vi "TAT_Start.vi"(8 "error In":errorcluster) -> (0 "error out":errorcluster)   [LabVIEW 2017]
uses:
  <vilib>/Utility/error.llb/DialogType.ctl
  Controls/Ass. Loop Control.ctl
  <vilib>/addons/database/Connection.llb/Conn ObjectReference.ctl
  227c0874-5cf7-40bb-b9d2-311cfb67fe7f.vi
  Global/Global 1.vi
  <vilib>/Instr/_visa.llb/VISA Configure Serial Port (Instr).vi
  <vilib>/addons/database/NI_Database_API.lvlib
  <vilib>/Utility/config.llb/NI_LVConfig.lvlib
panel:
  out "12 4":bool
  out "EOL AUTO CYCLE STATUS:-":bool
  out "12 3":bool
  out "12 2":bool
  out "12":bool
  out "PLC STATUS:-":bool
  out "array":string[](array[string])
  out "LEAK UNIT RESULT 2":bool caption="LEAK RESULT:-"
  out "LEAK ACTUAL VALUE 2":string
  out "LEAK MAX 2":string
  out "LEAK MIN 2":string
  out "LEAK UNIT RESULT":bool caption="LEAK RESULT:-"
  out "LEAK ACTUAL VALUE":string
  out "LEAK MAX":string
  out "LEAK MIN":string
  out "PREVIOUS BARCODE":string[](array[string])
  out "scanned":string
  out "Scanned Qyt":string
  out "PROJECT :-":string
  out "PACKAGE Qty":string
  out "TORISHI CODE:-":string
  out "PART No.:-":string
  in  "Stop":bool
  out "BARCODE STATION 2":string caption="BARCODE:-"
  out "RESULT STATION 1":bool caption="FINAL RESULT:-"
  out "USER:-":string
  out "PART NAME :-":string
  in  "ASS-Alarms":bool
  out "CYCLE STATUS STATION 1":string caption="CYCLE STATUS:-"
  out "DATE/TIME":string
  # "KAPSE SONS ROBOTICS\n& AUTOMATION"
  # "Nm"
  # "POKA-YOKE STATUS"
  # "LEAK TESTING PARAMETER"
  # "MIN"
  # "MAX"
  # "ACTUAL VALUE"
  # "RESULT"
  # "LEAK UNIT"
  # "LEAK PRESSURE"
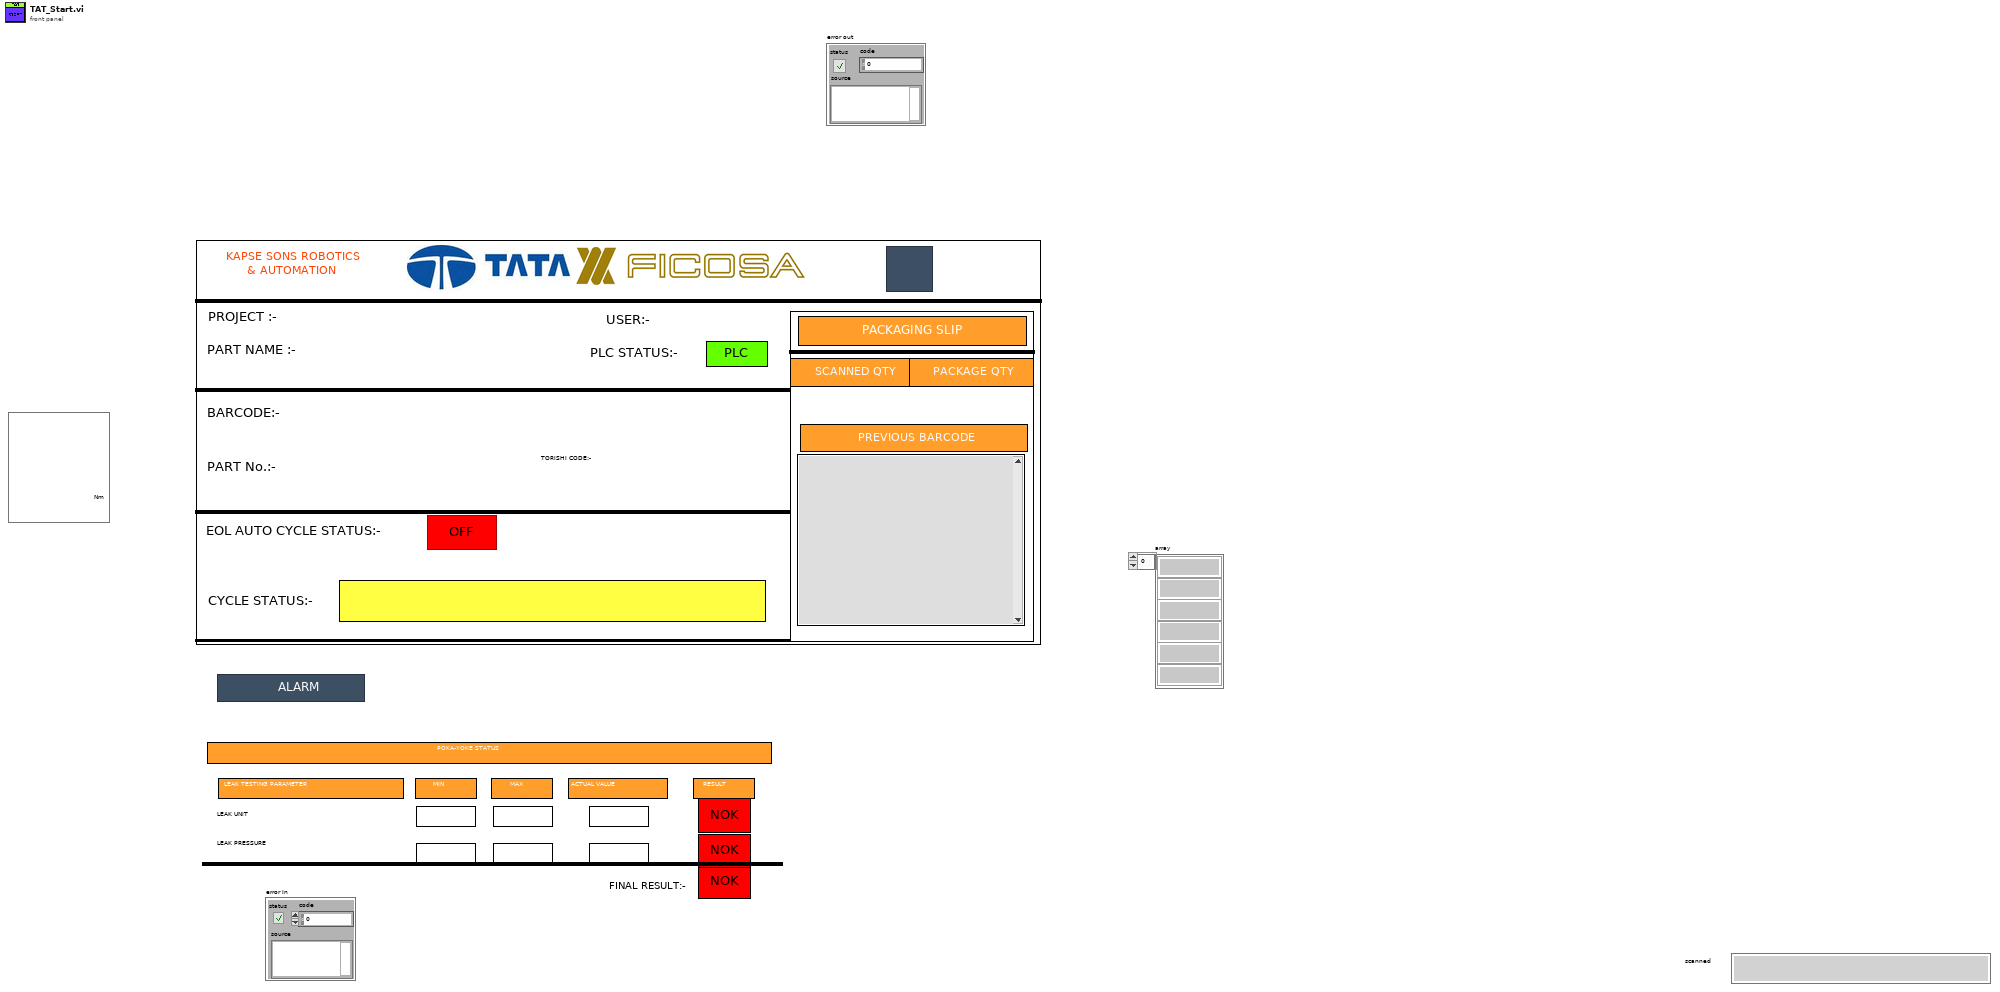
[diagram p1: front panel]
types:
  T1 = typedef "NI_Database_API.lvlib/Conn ObjectReference.ctl" = refnum<k1>
  T2 = cluster{"Varient number":u16, "Part name":string, "Barcode":string, "connection reference":T1, "Batch_Size":u16, "PART_NO":string, "TORISHI_CODE":string, "scanner com":refnum<visa-resource-name>, "Part Name List":string[], "Varient path":path, "Current Varient path":path, "Communication path":path, "PRN path":path, "printer":refnum<k5>, "Data_log_Path":path, "PREVIOUS Code":string[], "Printer IP add":string}
  T3 = typedef "Ass. Loop Control.ctl" = enum16{"Int2", "Package_Qty_Count", "GENERATE_QR_PRNT", "Cluster_update", "Waiting_for_scan", "barcode CHECK", "Int", "SaveReport ", "Barcode Print", "Start Cycle", "Wait", "Cycle End", "Stop"}
  T4 = typedef "DialogType.ctl" = u16
  T5 = enum32{"invalid app kind", "Development System", "Run Time System", "Student Edition", "Embedded LabVIEW", "Evaluation", "Custom"}
  T6 = typedef "NI_LVConfig.lvlib/Config Data RefNum.ctl" = refnum<k1>
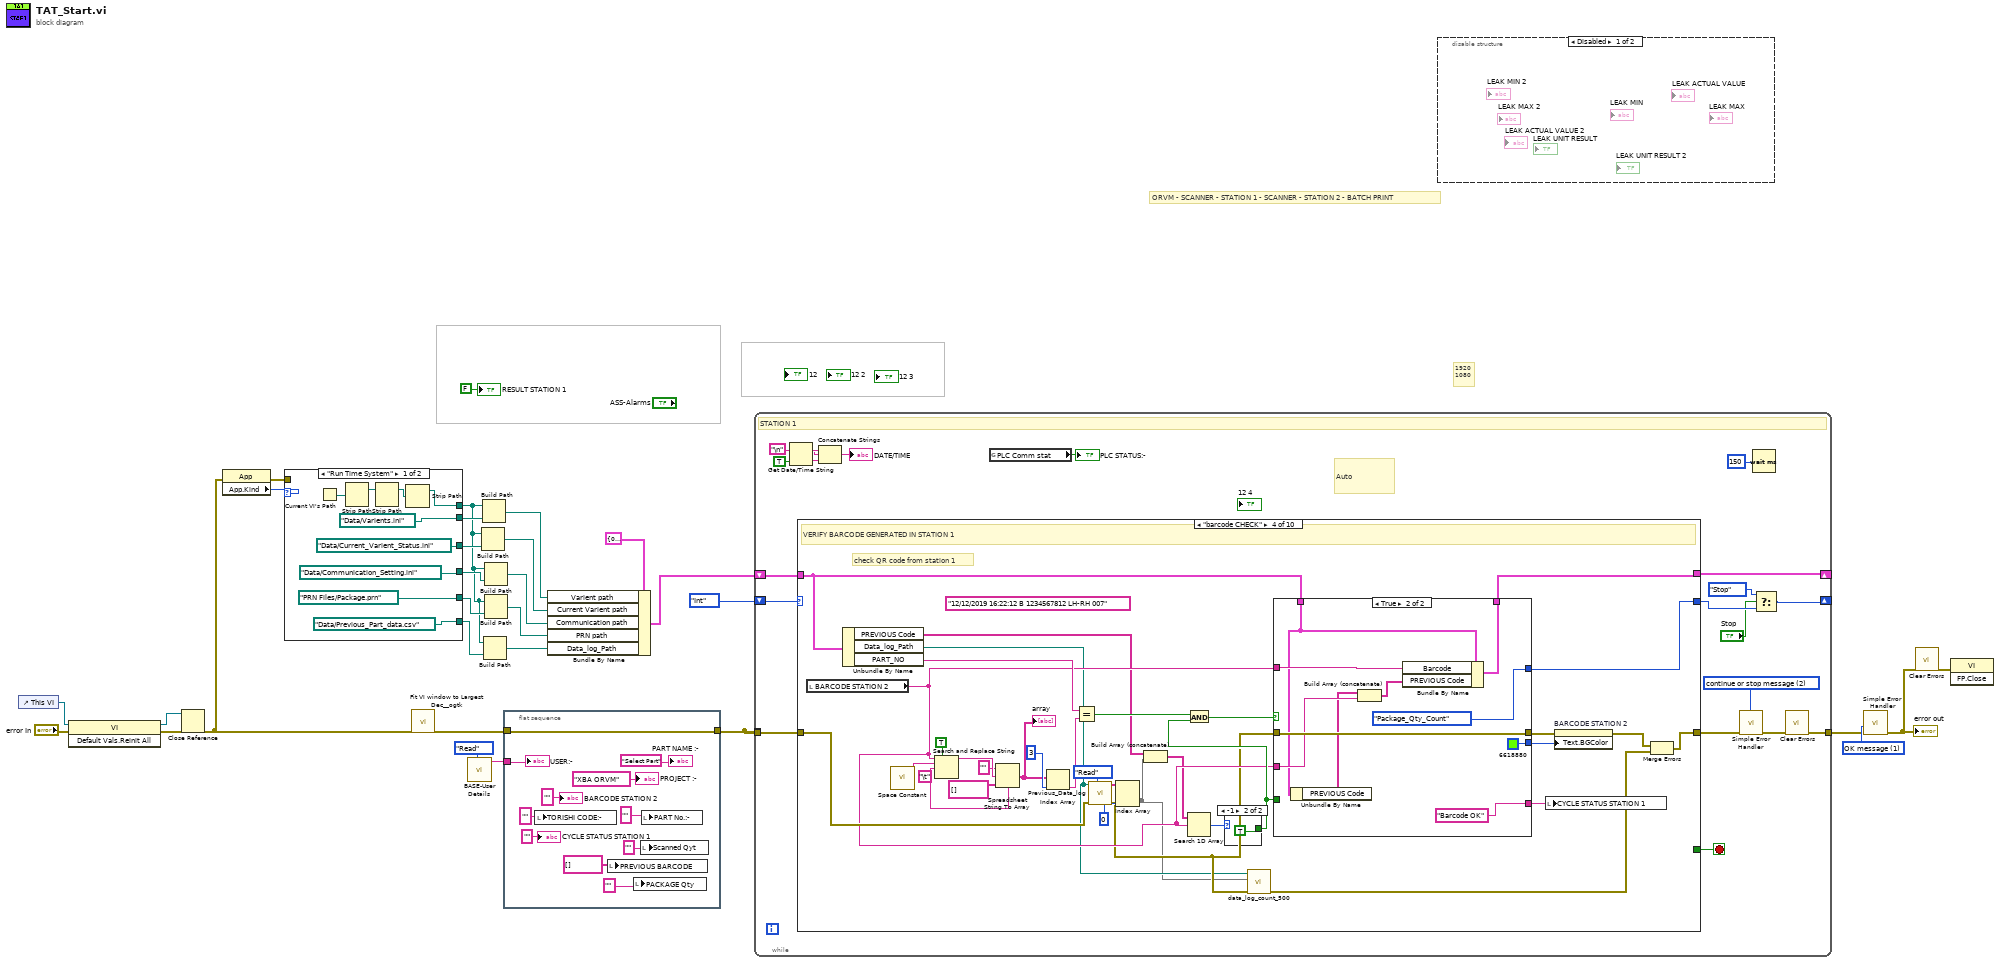
[diagram p0: block diagram]
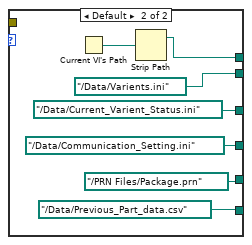
[diagram p2: hidden frame]
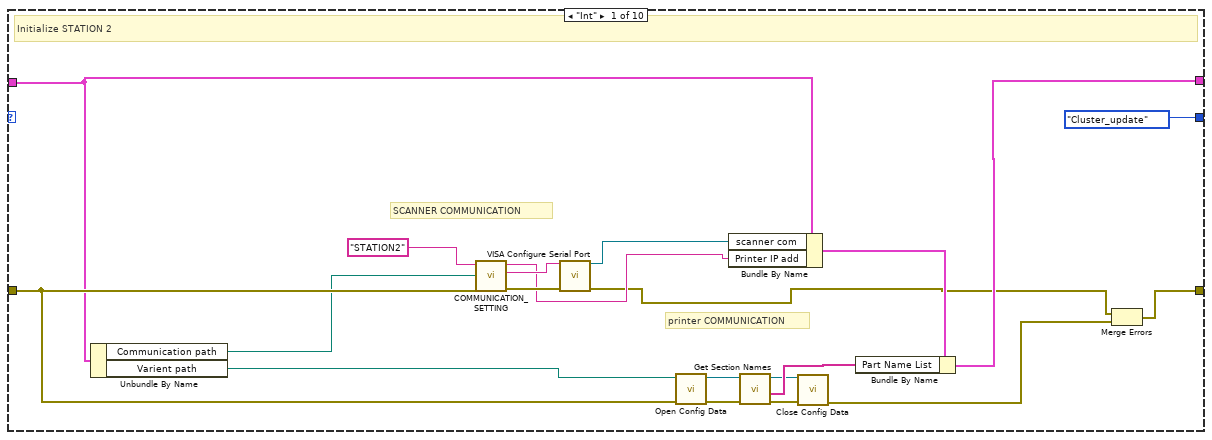
[diagram p4: hidden frame]
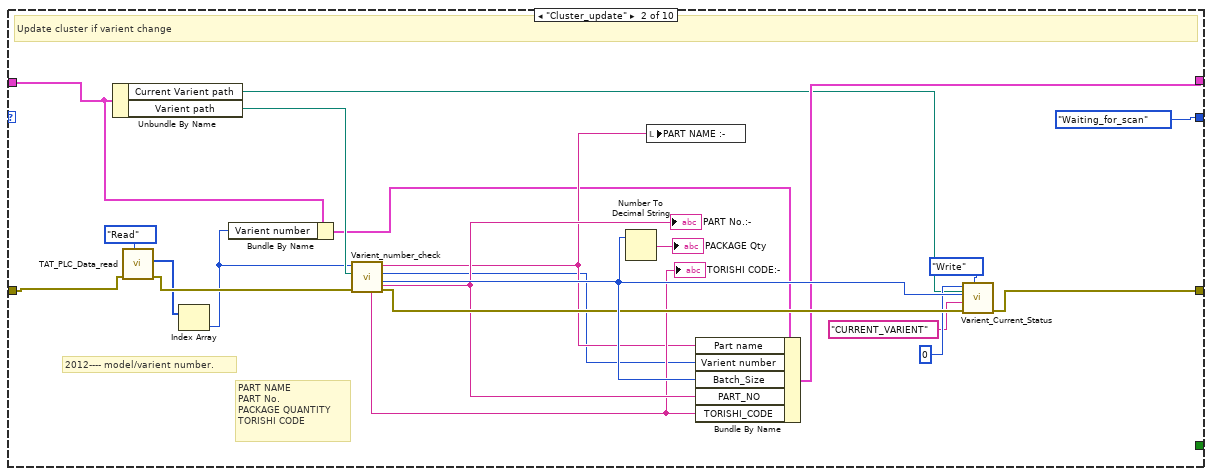
[diagram p5: hidden frame]
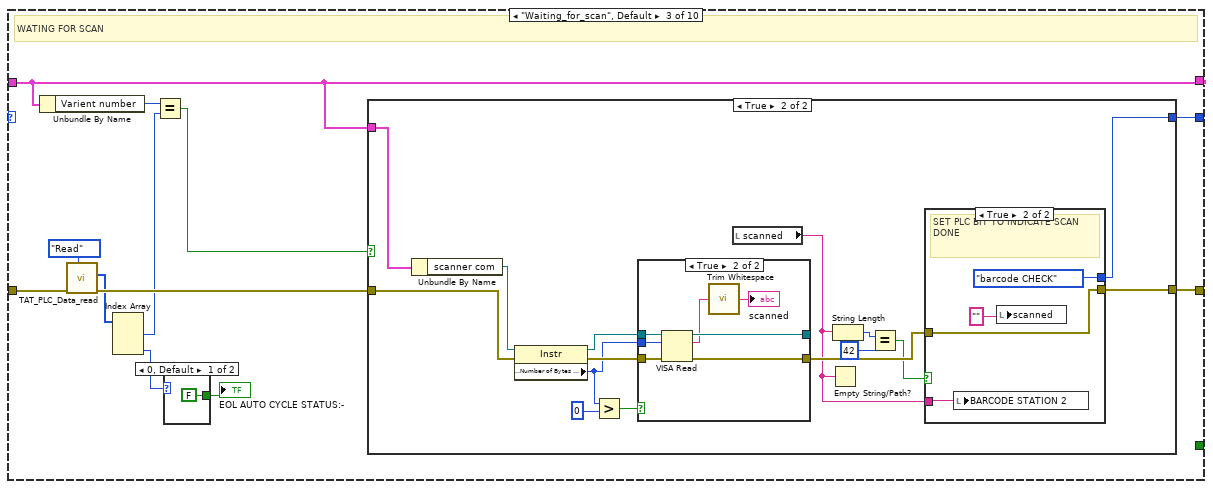
[diagram p6: hidden frame]
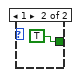
[diagram p7: hidden frame]
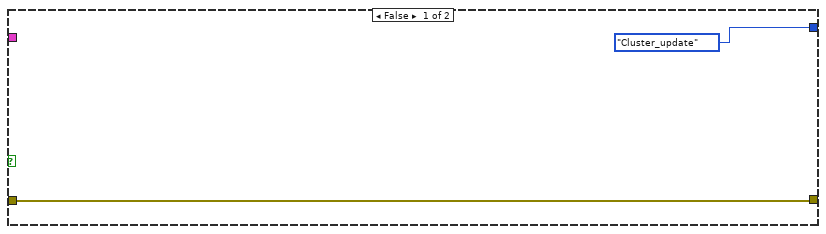
[diagram p8: hidden frame]
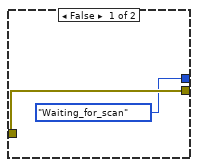
[diagram p10: hidden frame]
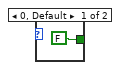
[diagram p11: hidden frame]
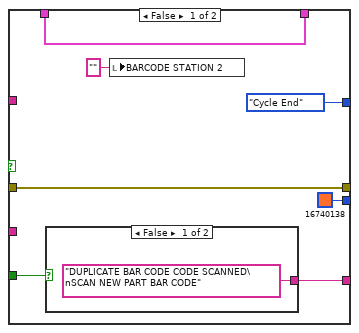
[diagram p12: hidden frame]
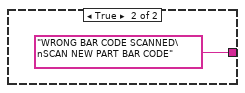
[diagram p13: hidden frame]
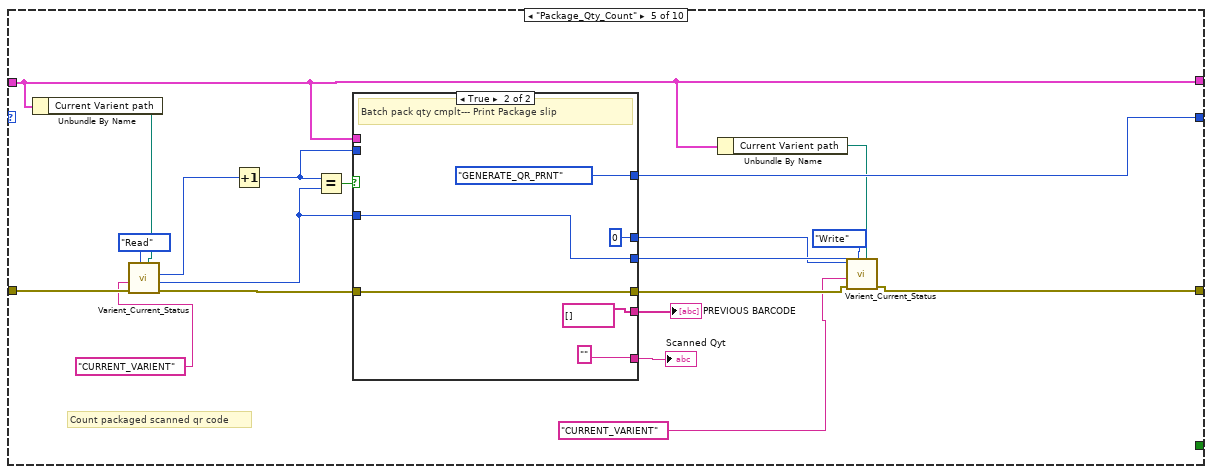
[diagram p14: hidden frame]
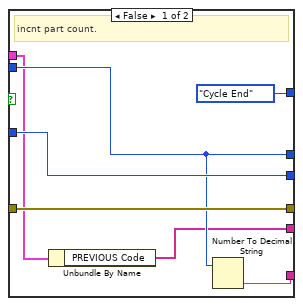
[diagram p15: hidden frame]
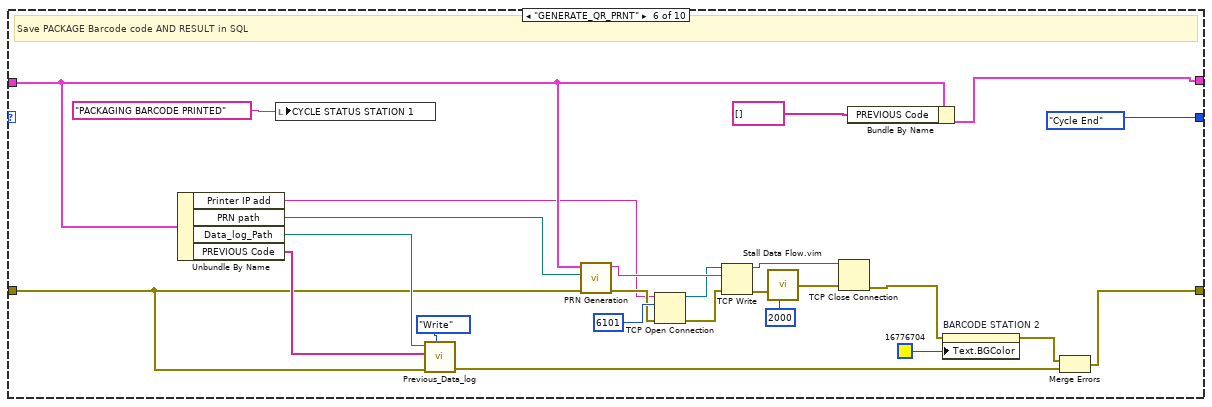
[diagram p16: hidden frame]
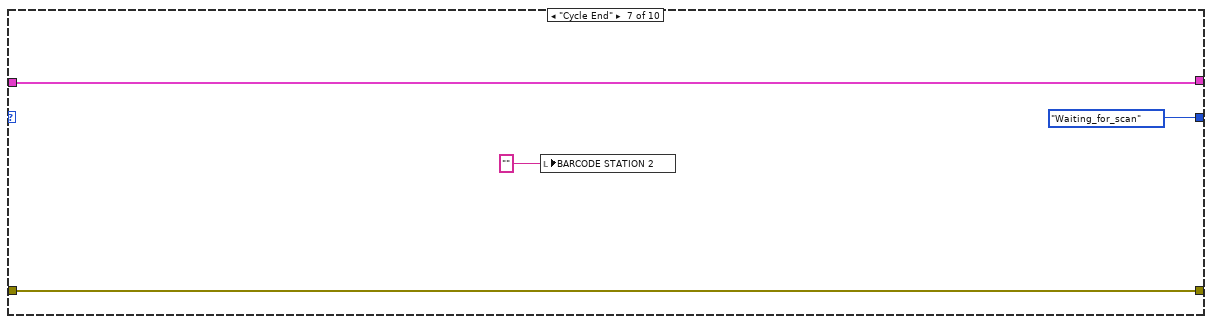
[diagram p17: hidden frame]
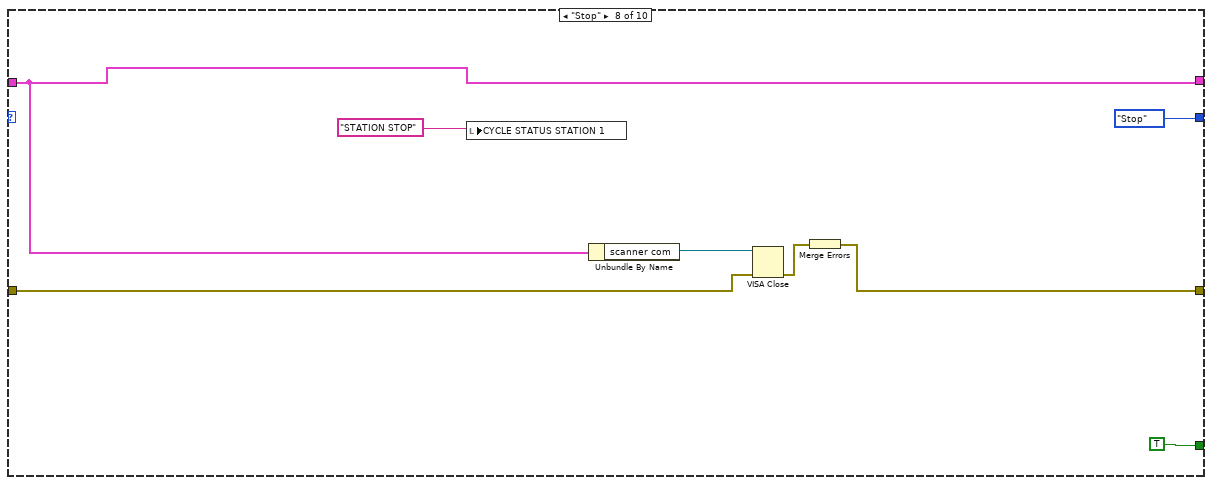
[diagram p18: hidden frame]
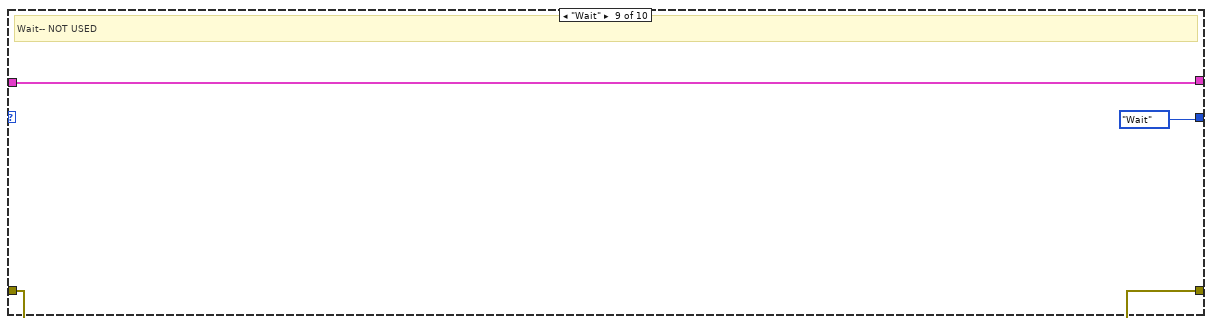
[diagram p19: hidden frame]
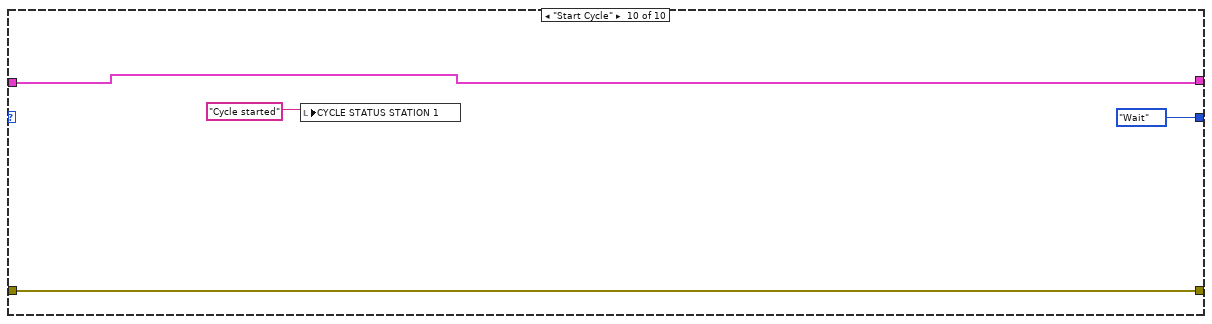
[diagram p20: hidden frame]
diagram:
  w20 = T4 1 items=["no dialog", "OK message", "continue or stop message", "OK message + warnings", "continue/stop + warnings"] ("type of dialog (OK msg:1)")
  # "1920\n1080"
  # "ORVM - SCANNER - STATION 1 - SCANNER - STATION 2 - BATCH PRINT"
  n1 = control-ref of="This VI"() -> (w30:refnum<vi>)
  n2 = invoke class="VI" method="Default Vals.Reinit All"(reference=w30, error in="error In") -> (reference out=w27:refnum<vi>, error out=w28:errorcluster)  [unwired: 1 in, 1 out]
  n3 = Close Reference(reference=w27, error in (no error)=w28) -> (error out=w4:errorcluster)
  n4 = property class="App"(error in=w4) -> (error out=w7:errorcluster, "App.Kind"=w16:T5)  [unwired: 1 in, 1 out]
  n5 = case shown="\"Run Time System\"" w16 {
    tunnel: [path "Data/Varients.ini" ("path") path "../Data/Varients.ini" ("path")] -> w15
    tunnel: [w35 w44] -> w5
    tunnel: [path "Data/Current_Varient_Status.ini" ("path") path "../Data/Current_Varient_Status.ini" ("path")] -> w12
    tunnel: [path "Data/Communication_Setting.ini" ("path") path "../Data/Communication_Setting.ini" ("path")] -> w11
    tunnel: [path "PRN Files/Package.prn" ("path") path "../PRN Files/Package.prn" ("path")] -> w9
    tunnel: w7 -> [_ _]
    tunnel: [path "Data/Previous_Part_data.csv" ("path") path "../Data/Previous_Part_data.csv" ("path")] -> w1
    frame "Run Time System" {
      n6 = Current VI's Path() -> (path=w38:path)
      n7 = Strip Path(path=w38) -> (stripped path=w37:path)  [unwired: 1 out]
      n8 = Strip Path(path=w37) -> (stripped path=w36:path)  [unwired: 1 out]
      n9 = Strip Path(path=w36) -> (stripped path=w35:path)  [unwired: 1 out]
    }
    frame Default {
      n10 = Current VI's Path() -> (path=w45:path)
      n11 = Strip Path(path=w45) -> (stripped path=w44:path)  [unwired: 1 out]
    }
  }
  n12 = call <userlib>:"Fit VI window to Largest Dec__ogtk.vi"("error in (no error)"=w4) -> ("error out"=w26:errorcluster)  [unwired: 5 in, 1 out]
  n13 = call "BASE-User Details.vi"("Enum"=enum16{"Read", "Write"}."Read") -> ("User Name Out"=w21:string)  [unwired: 9 in, 1 out]
  n14 = Build Path(base path=w5, name or relative path=w12) -> (appended path=w13:path)
  n15 = Build Path(base path=w5, name or relative path=w15) -> (appended path=w14:path)
  n16 = Build Path(base path=w5, name or relative path=w1) -> (appended path=w6:path)
  n17 = Build Path(base path=w5, name or relative path=w11) -> (appended path=w10:path)
  n18 = Build Path(base path=w5, name or relative path=w9) -> (appended path=w8:path)
  n19 = flat-sequence {
    tunnel: [w57] -> w18
    tunnel: w26 -> [w57]
    tunnel: w21 -> [w56]
    frame #0 {
      n20 = local write "TORISHI CODE:-"("") -> ()
      n21 = local write "PREVIOUS BARCODE"(string[] []) -> ()
      n22 = local write "PACKAGE Qty"("") -> ()
      n23 = local write "Scanned Qyt"("") -> ()
      n24 = local write "PART No.:-"("") -> ()
      "USER:-" <- w56
      "PART NAME :-" <- "Select Part"
      "PROJECT :-" <- "XBA ORVM" ("PROJECT")
      "BARCODE STATION 2" <- ""
      "CYCLE STATUS STATION 1" <- ""
    }
  }
  n25 = Bundle By Name(cluster=T2 {"Varient number"=0, "Part name"="", "Barcode"="", "connection reference"=refnum, "Batch_Size"=0, "PART_NO"="", "TORISHI_CODE"="", "scanner com"="", "Part Name List"=[], "Varient path"=path "", "Current Varient path"=path "", "Communication path"=path "", "PRN path"=path "", "printer"=refnum, "Data_log_Path"=path "", "PREVIOUS Code"=[], "Printer IP add"=""}, "Varient path"=w14, "Current Varient path"=w13, "Communication path"=w10, "PRN path"=w8, "Data_log_Path"=w6) -> (w2:T2)
  n26 = while {
    tunnel: w18 -> [_]
    shift-right: [w66] -> _
    shift-left: Ass._Loop_Control."Int" ("Enum") -> [w71]
    tunnel: w18 -> [w70]
    shift-right: [w68] -> _
    shift-left: w2 -> [w69]
    tunnel: [w59] -> w17
    stop <- w58 stop-if-true
    w63 = T4 2 items=["no dialog", "OK message", "continue or stop message", "OK message + warnings", "continue/stop + warnings"] ("type of dialog (OK msg:1)")
    # "Auto"
    # "STATION 1"
    n27 = Get Date/Time String(want seconds? (F)=TRUE) -> (date string=w75:string, time string=w74:string)  [unwired: 2 in]
    n28 = case shown="\"barcode CHECK\"" w71 {
      tunnel: [Ass._Loop_Control."Cluster_update" ("Enum") Ass._Loop_Control."Waiting_for_scan" ("Enum") w130 w174 w228 Ass._Loop_Control."Cycle End" ("Enum") Ass._Loop_Control."Waiting_for_scan" ("Enum") Ass._Loop_Control."Stop" ("Enum") Ass._Loop_Control."Wait" ("Enum") Ass._Loop_Control."Wait" ("Enum")] -> w65
      tunnel: [w84 w109 w125 w196 w220 w272 w280 w285 w292 w293] -> w68
      tunnel: [w83 w110 w131 w171 w233 w264 w278 w286 w290 w294] -> w62
      tunnel: w70 -> [w93 w103 w128 w178 w239 w266 w278 w283 w290 w294]
      tunnel: w69 -> [w92 w99 w125 w197 w220 w261 w280 w285 w292 w293]
      tunnel: [_ _ _ _ _ _ _ TRUE _ _] -> w58
      frame "Int" {
        # "printer COMMUNICATION"
        # "SCANNER COMMUNICATION"
        # "Initialize STATION 2"
        n29 = Unbundle By Name(w92) -> ("Communication path"=w81:path, "Varient path"=w82:path)
        n30 = call "COMMUNICATION_SETTING.vi"("communication path"=w81, "error in"=w93, "STATION"="STATION2") -> ("error out"=w96:errorcluster, "SCAN_COM"=w94:string, "PRINT_COM"=w80:string)  [unwired: 6 in]
        n31 = call-poly "VISA Configure Serial Port"("VISA resource name"=w94, "error in (no error)"=w96) -> ("VISA resource name out"=w78:refnum<visa-resource-name>, "error out"=w79:errorcluster)  [unwired: 12 in]
        n32 = call <vilib>:"Open Config Data.vi"("error in (no error)"=w93, "configuration file path"=w82) -> ("error out"=w89:errorcluster, "refnum"=w90:T6)  [unwired: 7 in, 1 out]
        n33 = Bundle By Name(cluster=w92, "scanner com"=w78, "Printer IP add"=w80) -> (w85:T2)
        n34 = call <vilib>:"Get Section Names.vi"("error in (no error)"=w89, "refnum"=w90) -> ("error out"=w88:errorcluster, "section names"=w91:string[], "refnum out"=w87:T6)  [unwired: 7 in]
        n35 = call <vilib>:"Close Config Data.vi"("error in (no error)"=w88, "refnum"=w87) -> ("error out"=w86:errorcluster)  [unwired: 8 in, 1 out]
        n36 = Bundle By Name(cluster=w85, "Part Name List"=w91) -> (w84:T2)
        n37 = Merge Errors(w79, w86) -> (w83:errorcluster)
      }
      frame "Cluster_update" {
        # "2012---- model/varient number."
        # "PART NAME\nPART No.\nPACKAGE QUANTITY\nTORISHI CODE"
        # "Update cluster if varient change"
        n38 = Unbundle By Name(w99) -> ("Current Varient path"=w105:path, "Varient path"=w106:path)
        n39 = call "TAT_PLC_Data_read.vi"("Enum"=enum16{"Read", "Write"}."Read", "error in (no error)"=w103) -> ("error out"=w102:errorcluster, "Array 2"=w101:u16[])  [unwired: 8 in]
        n40 = Index Array(array=w101) -> (element=w100:u16)  [unwired: 1 in]
        n41 = Bundle By Name(cluster=w99, "Varient number"=w100) -> (w98:T2)
        n42 = call "Varient_number_check.vi"("error in"=w102, "Varient path"=w106, "Varient No."=w100) -> ("error out"=w118:errorcluster, "Batch Size"=w119:i32, "Varient Number"=w113:i32, "Part Name"=w114:string, "PART_NO"=w117:string, "TORISHI_CODE"=w116:string)  [unwired: 3 in]
        "PART No.:-" <- w117
        "TORISHI CODE:-" <- w116
        n43 = Number To Decimal String(number=w119) -> (decimal integer string=→"PACKAGE Qty":string)  [unwired: 1 in]
        n44 = local write "PART NAME :-"(w114) -> ()
        n45 = Bundle By Name(cluster=w98, "Part name"=w114, "Varient number"=w113, "Batch_Size"=w119, "PART_NO"=w117, "TORISHI_CODE"=w116) -> (w109:T2)
        n46 = call "Varient_Current_Status.vi"("Currenrt Varient path"=w105, "Enum"=enum16{"Write", "Read"}."Write", "error in"=w118, "AUTO/MANUAL"="CURRENT_VARIENT", "Batch Size"=w119, "Varient count"=0) -> ("error out"=w110:errorcluster)  [unwired: 3 in, 2 out]
      }
      frame "Waiting_for_scan", Default {
        # "WATING FOR SCAN"
        n47 = Unbundle By Name(w125) -> ("Varient number"=w124:u16)
        n48 = call "TAT_PLC_Data_read.vi"("Enum"=enum16{"Read", "Write"}."Read", "error in (no error)"=w128) -> ("error out"=w127:errorcluster, "Array 2"=w126:u16[])  [unwired: 8 in]
        n49 = Index Array(array=w126) -> (element #1=w123:u16, element #3=w121:u16)  [unwired: 3 in, 1 out]
        n50 = Equal?(x=w124, y=w123) -> (x = y?=w122:bool)
        n51 = case shown="0, Default" w121 {
          tunnel: [FALSE TRUE] -> w120
          frame 0, Default {
          }
          frame 1 {
          }
        }
        "EOL AUTO CYCLE STATUS:-" <- w120
        n52 = case shown="True" w122 {
          tunnel: [w135 w147] -> w131
          tunnel: [Ass._Loop_Control."Cluster_update" ("Enum") w146] -> w130
          tunnel: w127 -> [w135 w137]
          tunnel: w125 -> [_ w136]
          frame False {
          }
          frame True {
            n53 = Unbundle By Name(w136) -> ("scanner com"=w145:refnum<visa-resource-name>)
            n54 = property class="Instr"(reference=w145, error in=w137) -> (reference out=w150:refnum<visa-resource-name>, error out=w149:errorcluster, "Serial Settings:Number of Bytes at Serial Port"=w144:u32)
            n55 = Greater?(x=w144, y=u32 0) -> (0:w143:bool)
            n56 = case shown="True" w143 {
              tunnel: w150 -> [w152 w159]
              tunnel: w149 -> [w151 w158]
              tunnel: w144 -> [_ w157]
              tunnel: [w152 w156] -> _
              tunnel: [w151 w153] -> w148
              frame False {
              }
              frame True {
                n57 = VISA Read(VISA resource name=w159, byte count=w157, error in (no error)=w158) -> (VISA resource name out=w156:refnum<visa-resource-name>, read buffer=w154:string, error out=w153:errorcluster)  [unwired: 1 out]
                n58 = call <vilib>:"Trim Whitespace.vi"("string"=w154) -> ("trimmed string"=→"scanned":string)  [unwired: 1 in]
              }
            }
            n59 = local read "scanned"() -> (w141:string)
            n60 = Empty String/Path?(string/path=w141) -> ()  [unwired: 1 out]
            n61 = String Length(string=w141) -> (length=w140:i32)
            n62 = Equal?(x=w140, y=42) -> (x = y?=w138:bool)
            n63 = case shown="True" w138 {
              tunnel: w148 -> [w161 w165]
              tunnel: [w161 w165] -> w147
              tunnel: w141 -> [_ w164]
              tunnel: [Ass._Loop_Control."Waiting_for_scan" ("Enum") Ass._Loop_Control."barcode CHECK" ("Enum")] -> w146
              frame False {
              }
              frame True {
                # "SET PLC BIT TO INDICATE SCAN DONE"
                n64 = local write "BARCODE STATION 2"(w164) -> ()
                n65 = local write "scanned"("") -> ()
              }
            }
          }
        }
      }
      frame "barcode CHECK" {
        w192 = "\t"
        (unwired) "12/12/2019 16:22:12 B 1234567812 LH-RH 007" ("string")
        # "check QR code from station 1"
        # "VERIFY BARCODE GENERATED IN STATION 1"
        n66 = local read "BARCODE STATION 2"() -> (w175:string)
        n67 = Unbundle By Name(w197) -> ("PREVIOUS Code"=w168:string[], "Data_log_Path"=w169:path, "PART_NO"=w188:string)
        n68 = call <vilib>:"Space Constant.vi"() -> ("String"=w195:string)
        n69 = Search and Replace String(replace all?=TRUE ("replace all? (F)"), input string=w175, search string=w195, replace string=w192) -> (result string=w193:string)  [unwired: 4 in, 3 out]
        n70 = Spreadsheet String To Array(delimiter (Tab)=w192, format string="", spreadsheet string=w193, array type (2D Dbl)=string[] []) -> (array=w184:string[])
        "array" <- w184
        n71 = Index Array(array=w184, index=3) -> (element=w187:string)
        n72 = Equal?(x=w188, y=w187) -> (x = y?=w186:bool)
        n73 = call "Previous_Data_log.vi"(7:enum16{"Write", "Read"}."Read", "error in (no error)"=w178, "file path (dialog if empty)"=w169) -> ("error out"=w173:errorcluster, "all rows"=w181:string[][])  [unwired: 7 in]
        n74 = Index Array(array=w181, index (col)=0 ("disabled index (col)")) -> (element=w167:string[])  [unwired: 1 in]
        n75 = Build Array (concatenate)(w168, w167) -> (w166:string[])
        n76 = Search 1D Array(1D array=w166, element=w175) -> (index of element=w182:i32)  [unwired: 1 in]
        n77 = case shown="-1" w182 {
          tunnel: [FALSE TRUE] -> w177
          frame 0, Default {
          }
          frame -1 {
          }
        }
        n78 = And(x=w186, y=w177) -> (x .and. y?=w185:bool)
        n79 = call "data_log_count_500.vi"("error in (no error)"=w173, "All data"=w167, "file path (dialog if empty)"=w169) -> ("error out"=w170:errorcluster)  [unwired: 8 in]
        n80 = case shown="True" w185 {
          tunnel: [w207 "Barcode OK" ("Cycle Status")] -> w198
          tunnel: w197 -> [w206 w212]
          tunnel: [w206 w218] -> w196
          tunnel: w175 -> [_ w217]
          tunnel: [u32 16740138 u32 6618880] -> w183
          tunnel: w177 -> [w201 _]
          tunnel: w173 -> [w204 w215]
          tunnel: [w204 w215] -> w176
          tunnel: w175 -> [_ w213]
          tunnel: [Ass._Loop_Control."Cycle End" ("Enum") Ass._Loop_Control."Package_Qty_Count" ("Enum")] -> w174
          frame False {
            n81 = case shown="False" w201 {
              tunnel: ["DUPLICATE BAR CODE CODE SCANNED\nSCAN NEW PART BAR CODE" ("Cycle Status") "WRONG BAR CODE SCANNED\nSCAN NEW PART BAR CODE" ("Cycle Status")] -> w207
              frame False {
              }
              frame True {
              }
            }
            n82 = local write "BARCODE STATION 2"("" ("BARCODE STATION 2")) -> ()
          }
          frame True {
            n83 = Unbundle By Name(w212) -> ("PREVIOUS Code"=w211:string[])
            n84 = Build Array (concatenate)(w211, w213) -> (w214:string[])
            n85 = Bundle By Name(cluster=w212, "Barcode"=w217, "PREVIOUS Code"=w214) -> (w218:T2)
          }
        }
        n86 = local write "CYCLE STATUS STATION 1"(w198) -> ()
        n87 = property on="BARCODE STATION 2" class="Str"(error in=w176, "Text.BGColor"=w183) -> (error out=w172:errorcluster)  [unwired: 1 in, 1 out]
        n88 = Merge Errors(w172, w170) -> (w171:errorcluster)
      }
      frame "Package_Qty_Count" {
        # "Count packaged scanned qr code"
        n89 = Unbundle By Name(w220) -> ("Current Varient path"=w224:path)
        n90 = call "Varient_Current_Status.vi"("Currenrt Varient path"=w224, "Enum"=enum16{"Write", "Read"}."Read", "error in"=w239, "AUTO/MANUAL"="CURRENT_VARIENT") -> ("error out"=w237:errorcluster, "Batch Size"=w231:i32, "Varient Count"=w236:i32)  [unwired: 5 in]
        n91 = Increment(x=w236) -> (x+1=w223:i32)
        n92 = Equal?(x=w223, y=w231) -> (x = y?=w235:bool)
        n93 = case shown="True" w235 {
          tunnel: [w246 w252] -> w232
          tunnel: w237 -> [w246 w252]
          tunnel: w223 -> [w242 _]
          tunnel: w231 -> [w245 w251]
          tunnel: [w245 w251] -> w230
          tunnel: [w242 0] -> w229
          tunnel: [Ass._Loop_Control."Cycle End" ("Enum") Ass._Loop_Control."GENERATE_QR_PRNT" ("Enum")] -> w228
          tunnel: [w240 string[] [] ("PREVIOUS BARCODE")] -> w222
          tunnel: [w243 ""] -> w221
          tunnel: w220 -> [w241 _]
          frame False {
            # "incnt part count."
            n94 = Unbundle By Name(w241) -> ("PREVIOUS Code"=w240:string[])
            n95 = Number To Decimal String(number=w242) -> (decimal integer string=w243:string)  [unwired: 1 in]
          }
          frame True {
            # "Batch pack qty cmplt--- Print Package slip"
          }
        }
        "PREVIOUS BARCODE" <- w222
        "Scanned Qyt" <- w221
        n96 = Unbundle By Name(w220) -> ("Current Varient path"=w225:path)
        n97 = call "Varient_Current_Status.vi"("Currenrt Varient path"=w225, "Enum"=enum16{"Write", "Read"}."Write", "error in"=w232, "AUTO/MANUAL"="CURRENT_VARIENT", "Batch Size"=w230, "Varient count"=w229) -> ("error out"=w233:errorcluster)  [unwired: 3 in, 2 out]
      }
      frame "GENERATE_QR_PRNT" {
        # "Save PACKAGE Barcode code AND RESULT in SQL"
        n98 = Unbundle By Name(w261) -> ("Printer IP add"=w253:string, "PRN path"=w271:path, "Data_log_Path"=w268:path, "PREVIOUS Code"=w267:string[])
        n99 = local write "CYCLE STATUS STATION 1"("PACKAGING BARCODE PRINTED" ("Cycle Status")) -> ()
        n100 = call "Previous_Data_log.vi"(7:enum16{"Write", "Read"}."Write", "error in (no error)"=w266, "Data IN"=w267, "file path (dialog if empty)"=w268) -> ("error out"=w263:errorcluster)  [unwired: 6 in, 1 out]
        n101 = call "PRN Generation.vi"("error in (no error)"=w266, "PRN path"=w271, "Cluster"=w261) -> ("error out"=w259:errorcluster, "PRN to Print"=w275:string)  [unwired: 7 in]
        n102 = TCP Open Connection(address=w253, remote port or service name=u16 6101, error in (no error)=w259) -> (connection ID=w257:refnum<k5>, error out=w258:errorcluster)  [unwired: 2 in]
        n103 = TCP Write(connection ID=w257, data in=w275, error in (no error)=w258) -> (connection ID out=w254:refnum<k5>, error out=w262:errorcluster)  [unwired: 1 in, 1 out]
        n104 = call "Stall Data Flow.vim"("value in"=w262, "milliseconds to wait"=u32 2000) -> ("value out"=w256:errorcluster)  [unwired: 1 out]
        n105 = TCP Close Connection(connection ID=w254, error in (no error)=w256) -> (error out=w255:errorcluster)  [unwired: 1 in, 1 out]
        n106 = Bundle By Name(cluster=w261, "PREVIOUS Code"=string[] []) -> (w272:T2)
        n107 = property on="BARCODE STATION 2" class="Str"(error in=w255, "Text.BGColor"=u32 16776704) -> (error out=w265:errorcluster)  [unwired: 1 in, 1 out]
        n108 = Merge Errors(w265, w263) -> (w264:errorcluster)
      }
      frame "Cycle End" {
        n109 = local write "BARCODE STATION 2"("" ("BARCODE STATION 2")) -> ()
      }
      frame "Stop" {
        n110 = local write "CYCLE STATUS STATION 1"("STATION STOP" ("Cycle Status")) -> ()
        n111 = Unbundle By Name(w285) -> ("scanner com"=w284:refnum<visa-resource-name>)
        n112 = VISA Close(VISA resource name=w284, error in (no error)=w283) -> (error out=w287:errorcluster)
        n113 = Merge Errors(w287) -> (w286:errorcluster)
      }
      frame "Wait" {
        # "Wait-- NOT USED"
      }
      frame "Start Cycle" {
        n114 = local write "CYCLE STATUS STATION 1"("Cycle started" ("Cycle Status")) -> ()
      }
    }
    n115 = Concatenate Strings(w75, "\n", w74) -> (→"DATE/TIME":string)
    n116 = global read "Global 1.vi" "PLC Comm stat"() -> (→"PLC STATUS:-":bool)
    n117 = call <vilib>:"Simple Error Handler.vi"("type of dialog (OK msg:1)"=w63, "error in (no error)"=w62) -> ("error out"=w60:errorcluster)  [unwired: 3 in, 4 out]
    n118 = Wait (ms)(milliseconds to wait=u32 150) -> ()  [unwired: 1 out]
    n119 = Select(t=Ass._Loop_Control."Stop" ("Enum"), s="Stop", f=w65) -> (s? t:f=w66:T3)
    n120 = call <vilib>:"Clear Errors.vi"("error in (no error)"=w60) -> ("error out"=w59:errorcluster)  [unwired: 5 in, 1 out]
  }
  n121 = disable-structure shown="Disabled" {
    frame Disabled {
    }
    frame Enabled {
    }
  }
  n122 = call <vilib>:"Simple Error Handler.vi"("type of dialog (OK msg:1)"=w20, "error in (no error)"=w17) -> ("error out"=w24:errorcluster)  [unwired: 3 in, 4 out]
  "error out" <- w24
  n123 = call <vilib>:"Clear Errors.vi"("error in (no error)"=w24) -> ("error out"=w23:errorcluster)  [unwired: 5 in, 1 out]
  n124 = invoke class="VI" method="FP.Close"(error in=w23) -> ()  [unwired: 2 in, 3 out]
  "RESULT STATION 1" <- FALSE ("want seconds? (F)")
